vi "SetUp.vi"(8 "error in (no error)":errorcluster, 11 "Prueba08 in":refnum<class "Prueba08.lvclass">) -> (0 "error out":errorcluster, 3 "Prueba08 out":refnum<class "Prueba08.lvclass">)   [LabVIEW 2019, in "Prueba08.lvclass"]
uses:
  Prueba08.lvclass
  Prueba08.lvclass/Prueba08.ctl
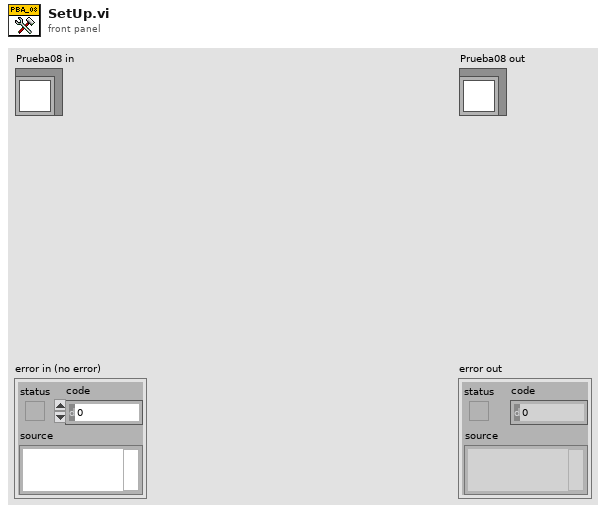
[diagram p1: front panel]
types:
  T1 = typedef "Prueba08.lvclass/BD.ctl" = cluster{"niv_presion_son_ref":dbl, "min_rango_ref":dbl, "max_rango_ref":dbl, "Incertidumbre":string[], "Tol +":string[], "Tol -":string[]}
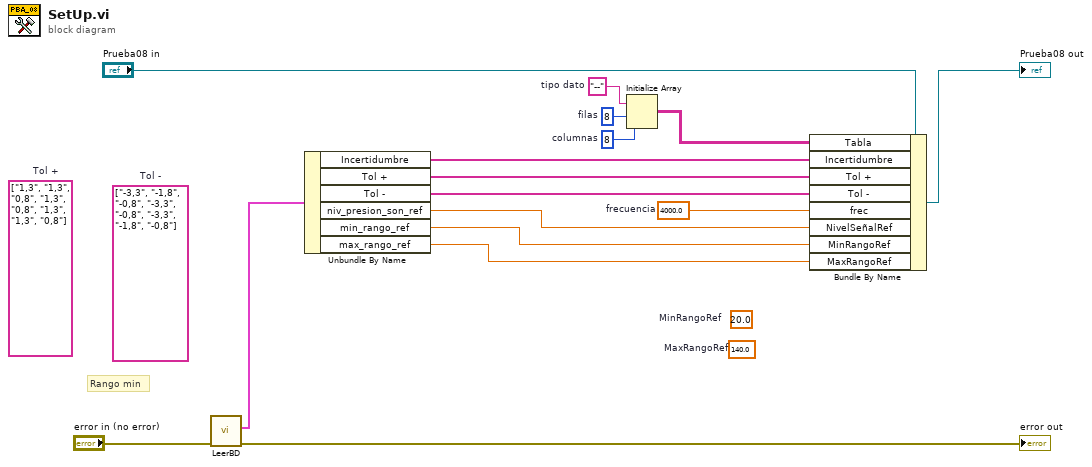
[diagram p0: block diagram]
diagram:
  (unwired) 140.0  # MaxRangoRef
  (unwired) 20.0  # MinRangoRef
  w15 = 4000.0  # frecuencia
  (unwired) string[] ["-3,3", "-1,8", "-0,8", "-3,3", "-0,8", "-3,3", "-1,8", "-0,8"]  # Tol -
  (unwired) string[] ["1,3", "1,3", "0,8", "1,3", "0,8", "1,3", "1,3", "0,8"]  # Tol +
  w13 = 8  # columnas
  w12 = 8  # filas
  w14 = "--"  # tipo dato
  # "Rango min"
  n1 = call "LeerBD.vi"("error in (no error)"="error in (no error)") -> ("error out"=→"error out":errorcluster, "BD"=w7:T1)  [unwired: 8 in, 1 out]
  n2 = Unbundle By Name(w7) -> ("Incertidumbre"=w6:string[], "Tol +"=w5:string[], "Tol -"=w4:string[], "niv_presion_son_ref"=w3:dbl, "min_rango_ref"=w2:dbl, "max_rango_ref"=w1:dbl)
  n3 = Initialize Array(w14, w12, w13) -> (w11:string[][])
  n4 = Bundle By Name(cluster="Prueba08 in", "Tabla"=w11, "Incertidumbre"=w6, "Tol +"=w5, "Tol -"=w4, "frec"=w15, "NivelSeñalRef"=w3, "MinRangoRef"=w2, "MaxRangoRef"=w1) -> (→"Prueba08 out":refnum<class "Prueba08.lvclass">)
